vi "SetExpOut.vi"(9 "Exp. in":refnum<vi>, 10 "ExposeOutMode":refnum<k24>, 11 "Digital in":refnum<vi>) -> ()   [LabVIEW 2019]
uses:
  Dependencies/PVCamNET.dll
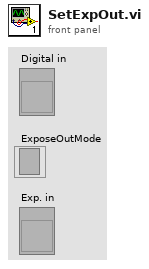
[diagram p1: front panel]
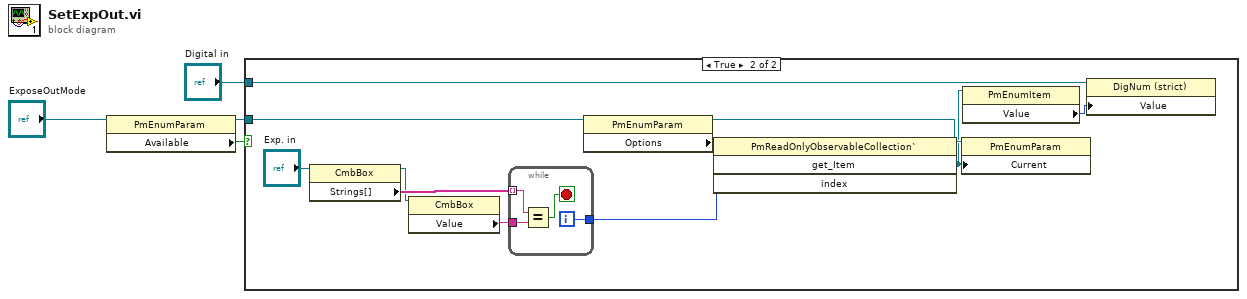
[diagram p0: block diagram]
diagram:
  n1 = property class="PmEnumParam"(reference="ExposeOutMode") -> (reference out=w2:refnum<k24>, "Available"=w3:bool)  [unwired: 1 in, 1 out]
  n2 = case shown="True" w3 {
    tunnel: w2 -> [_ w13]
    tunnel: "Digital in" -> [_ w7]
    frame False {
    }
    frame True {
      n3 = property class="CmbBox"(reference="Exp. in") -> (reference out=w6:refnum<vi>, "Strings[]"=w14:string[])  [unwired: 1 in, 1 out]
      n4 = property class="CmbBox"(reference=w6) -> ("Value"=w5:string)  [unwired: 1 in, 2 out]
      n5 = while {
        tunnel: w14 -> [w19] mode=indexing
        tunnel: [w17] -> w11
        tunnel: w5 -> [w16]
        i -> [w17]
        stop <- w18 stop-if-true
        n6 = Equal?(x=w19, y=w16) -> (x = y?=w18:bool)
      }
      n7 = property class="PmEnumParam"(reference=w13) -> (reference out=w10:refnum<k24>, "Options"=w12:refnum<k24>)  [unwired: 1 in, 1 out]
      n8 = invoke class="PmReadOnlyObservableCollection`" method="get_Item"(reference=w12, "index"=w11) -> ("get_Item"=w9:refnum<k24>)  [unwired: 2 in, 3 out]
      n9 = property class="PmEnumParam"(reference=w10, "Current"=w9) -> ()  [unwired: 1 in, 2 out]
      n10 = property class="PmEnumItem"(reference=w9) -> ("Value"=w8:i32)  [unwired: 1 in, 2 out]
      n11 = property class="DigNum (strict)"(reference=w7, "Value"=w8) -> ()  [unwired: 1 in, 2 out]
    }
  }
